vi "0p15mmSplit.vi"(1 "Est. Center":T1 {"U" format="%#.5g"; "X" format="%#.5g"; "Y" format="%#.5g"; "Z" format="%#.5g"}, 2 "Length":dbl=0.5 format="%#_13g", 3 "Direction":T1 {"U" format="%#.5g"; "X" format="%#.5g"; "Y" format="%#.5g"; "Z" format="%#.5g"}, 4 "RoughEdge":T1 {"U" format="%#.5g"; "X" format="%#.5g"; "Y" format="%#.5g"; "Z" format="%#.5g"}) -> (0 "Start":T1 {"U" format="%#.5g"; "X" format="%#.5g"; "Y" format="%#.5g"; "Z" format="%#.5g"})   [LabVIEW 2016]
uses:
  Control/Coordinate.ctl
  <vilib>/vision/NI_Vision_Development_Module.lvlib
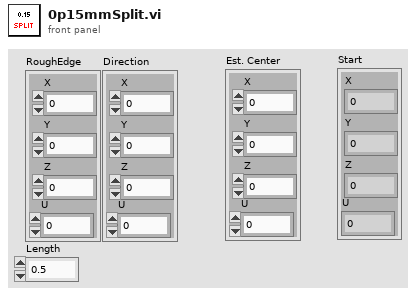
[diagram p1: front panel]
types:
  T1 = typedef "Coordinate.ctl" = cluster{"X":dbl, "Y":dbl, "Z":dbl, "U":dbl}
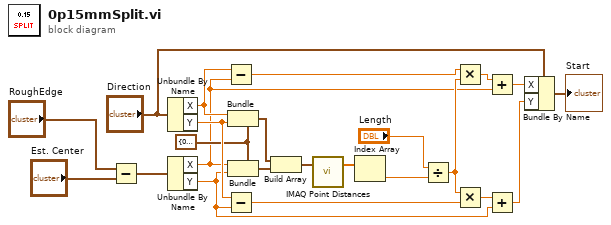
[diagram p0: block diagram]
diagram:
  w17 = cluster{"X":sgl, "Y":sgl} {"X"=0.0, "Y"=0.0}
  n1 = Subtract(x="RoughEdge", y="Est. Center") -> (x-y=w22:T1)
  n2 = Unbundle By Name("Direction") -> ("X"=w19:dbl, "Y"=w18:dbl)
  n3 = Unbundle By Name(w22) -> ("X"=w4:dbl, "Y"=w3:dbl)
  n4 = Subtract(x=w19, y=w4) -> (x-y=w10:dbl)
  n5 = Subtract(x=w18, y=w3) -> (x-y=w9:dbl)
  n6 = Bundle(cluster=w17, "X"=w19, "Y"=w18) -> (w16:cluster{"X":sgl, "Y":sgl})
  n7 = Bundle(cluster=w17, "X"=w4, "Y"=w3) -> (w15:cluster{"X":sgl, "Y":sgl})
  n8 = Build Array(w16, w15) -> (w14:cluster{"X":sgl, "Y":sgl}[])
  n9 = call "IMAQ Point Distances"("Points"=w14) -> ("Distances"=w12:sgl[])  [unwired: 4 in, 1 out]
  n10 = Index Array(array=w12) -> (element=w11:sgl)  [unwired: 1 in]
  n11 = Divide(x="Length", y=w11) -> (x/y=w8:dbl)
  n12 = Multiply(x=w10, y=w8) -> (x*y=w7:dbl)
  n13 = Multiply(x=w8, y=w9) -> (x*y=w2:dbl)
  n14 = Add(x=w7, y=w4) -> (x+y=w6:dbl)
  n15 = Add(x=w2, y=w3) -> (x+y=w5:dbl)
  n16 = Bundle By Name(cluster="Direction", "X"=w6, "Y"=w5) -> (→"Start":T1)
